vi "host_read_VISA.vi"() -> ()   [LabVIEW 2019]
uses:
  Program Files (x86)/National Instruments/LabVIEW 2019/examples/Instrument IO/Serial/support/Serial - Settings.ctl
  <vilib>/Platform/TimedLoop/XDataNode/timing_clust.ctl
  <vilib>/Platform/TimedLoop/XDataNode/nitl_modes.ctl
  <vilib>/Platform/TimedLoop/XDataNode/wakeup.ctl
  <vilib>/Instr/_visa.llb/VISA Configure Serial Port (Instr).vi
  <vilib>/Utility/file.llb/Write Delimited Spreadsheet (string).vi
  <vilib>/platform/TimedLoop/XDataNode/XDataNode.xnode
  <vilib>/Platform/TimedLoop/XDataNode/XDNodeRunTimeDep.lvlib
panel:
  in  "Data Read Period (ms)":i64=5
  out "data to write":string[](array[string])
  out "Date Formatted with Milliseconds":string
  out "LabVIEW TimeStamp":timestamp
  in  "file path (dialog if empty)":path=path "C:/Users/steve/Dropbox (MIT)/PhD Research/GPASS 2/Electronics/GPASS2-Electronics/Labview/GPASS 2/Data Files/serial/iros_serial.csv"
  in  "Channel Names":string[](array[string])=["Channel 1", "Channel 2", "Channel 3", "Channel 4", "Channel 5"]
  in  "Header Info":string[][](array[string])=[["Test Name", "Operator", "UUT"], ["Voltage", "National Instruments", "AA123"]]
  out "error out":errorcluster
  in  "stop":bool
  in  "End Read on Termination Character?":bool=TRUE
  in  "Serial Settings (read)":T1={"baud rate"=115200, "data bits"=8, "parity"=enum."None", "stop bits"=10, "flow control"=0} {"flow control" items=["None"=0, "XON/XOFF"=1, "RTS/CTS"=2, "DTR/DSR"=4]; "stop bits" items=["1.0"=10, "1.5"=15, "2.0"=20]; "data bits" min=5 max=8 step=1; "baud rate" items=["75"=75, "110"=110, "134"=134, "150"=150, "300"=300, "600"=600, "1200"=1200, "1800"=1800, "2400"=2400, "4800"=4800, "7200"=7200, "9600"=9600, "14400"=14400, "19200"=19200, "28800"=28800, "38400"=38400, "56000"=56000, "57600"=57600, "115200"=115200, "128000"=128000, "230400"=230400]}
  in  "VISA Resource (read)":refnum<visa-resource-name>="COM3"
  out "Read String":string
  out "bytes read":u32
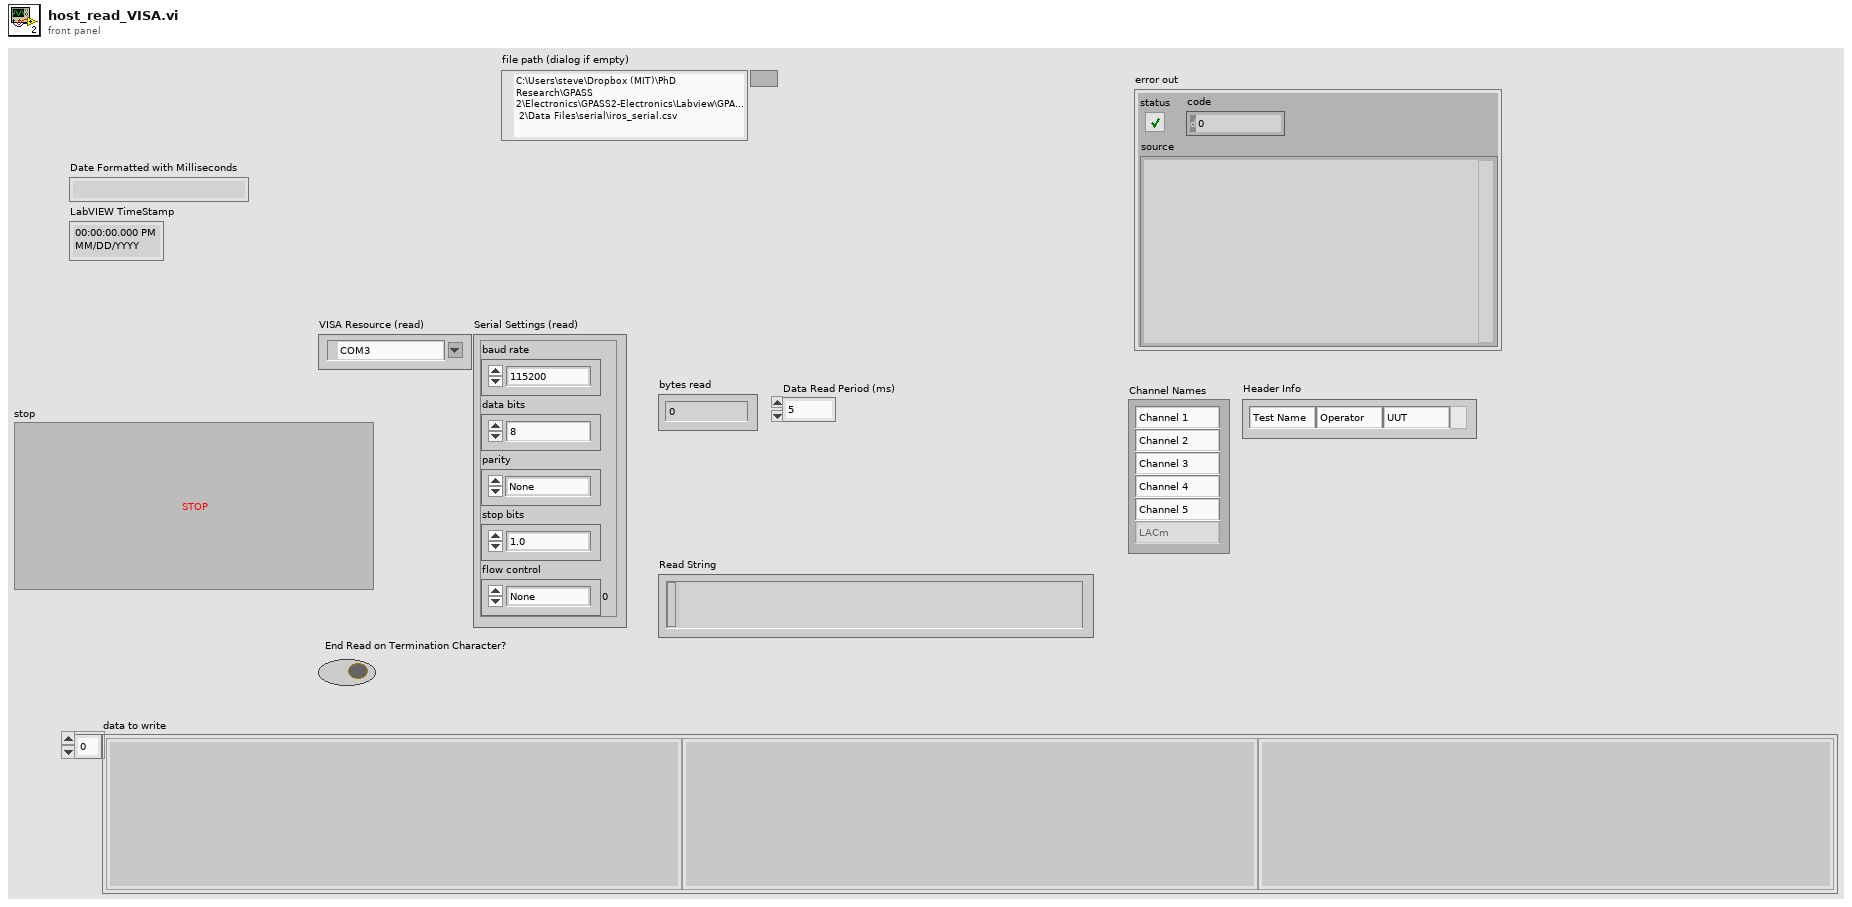
[diagram p1: front panel]
types:
  T1 = typedef "Serial - Settings.ctl" = cluster{"baud rate":u32, "data bits":u16, "parity":enum16{"None", "Odd", "Even", "Mark", "Space"}, "stop bits":u16, "flow control":u16}
  T2 = typedef "XDNodeRunTimeDep.lvlib/timing_clust.ctl" = cluster{"Expected End [f-1]":u64, "Actual End [f-1]":u64, "Finished Late? [f-1]":bool, "Expected End [i-1]":u64, "Actual End [i-1]":u64, "Finished Late? [i-1]":bool, "Expected Start [i]":u64, "Actual Start [i]":u64, "Expected Start [f]":u64, "Actual Start [f]":u64, "Source Name":string, "Structure Name":string, "Period":i64, "Deadline":i64, "Offset":i64, "Start":i64, "Priority":i32, "Timeout":i32, "Mode":T3, "Wakeup Reason":T4, "Error":errorcluster, "Source Type":string, "Secondary Source Type":string, "Global End Time":u64, "Global Start Time":u64, "Frame Duration":u64, "Iteration Duration":u64, "Assigned CPU":i32, "I/O Scan Engine Mode":u32}
  T3 = typedef "XDNodeRunTimeDep.lvlib/nitl_modes.ctl" = enum32{"No Change", "Process missed periods, maintain original phase", "Discard missed periods, maintain original phase", "Process missed periods, ignore original phase", "Discard missed periods, ignore original phase"}
  T4 = typedef "XDNodeRunTimeDep.lvlib/wakeup.ctl" = enum32{"Normal", "Aborted", "Asynchronous wakeup", "Timing source error", "Timed loop error", "Timeout"}
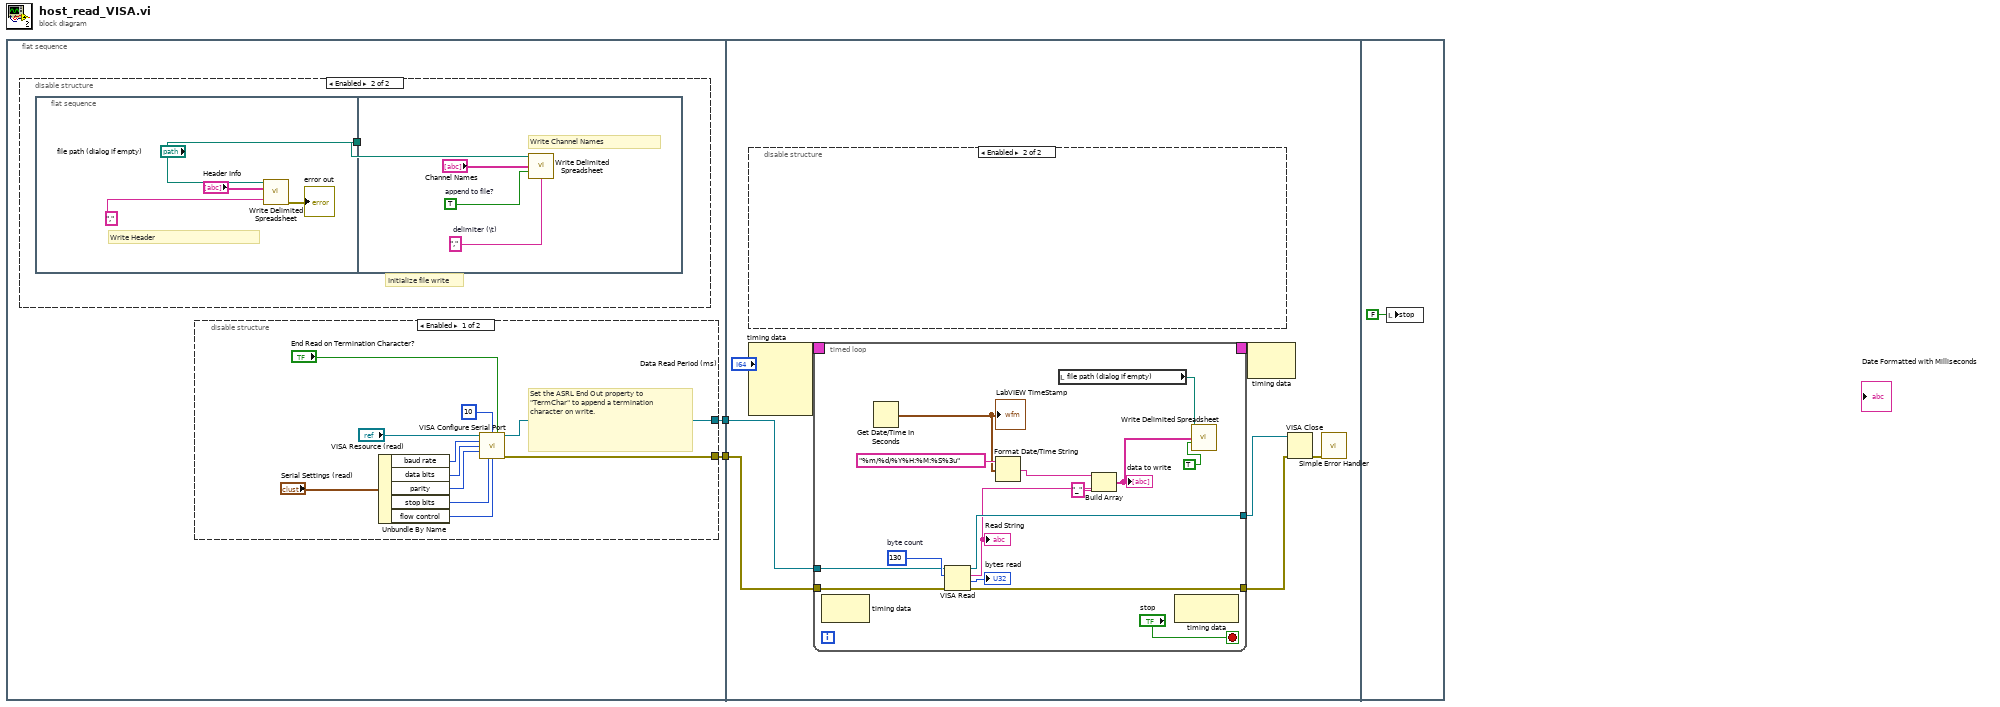
[diagram p0: block diagram]
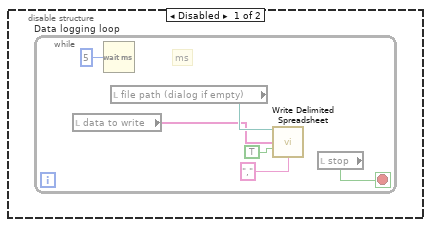
[diagram p4: hidden frame]
diagram:
  n1 = flat-sequence {
    tunnel: [w4] -> w2
    tunnel: [w3] -> w1
    tunnel: w2 -> [w27]
    tunnel: w1 -> [w26]
    frame #0 {
      n2 = disable-structure shown="Enabled" {
        frame Disabled {
        }
        frame Enabled {
          # "Initialize file write"
          n3 = flat-sequence {
            tunnel: ["file path (dialog if empty)"] -> w5
            tunnel: w5 -> [w10]
            frame #0 {
              # "Write Header"
              n4 = call-poly <vilib>:"Write Delimited Spreadsheet.vi"("file path (dialog if empty)"="file path (dialog if empty)", "2D data"="Header Info", "delimiter (\\t)"="," ("delimiter (\\t)")) -> ("error out"=→"error out":errorcluster)  [unwired: 11 in, 1 out]
            }
            frame #1 {
              w12 = TRUE  # append to file?
              w11 = ","  # delimiter (\t)
              # "Write Channel Names"
              n5 = call-poly <vilib>:"Write Delimited Spreadsheet.vi"("file path (dialog if empty)"=w10, "1D data"="Channel Names", "append to file? (new file:F)"=w12, "delimiter (\\t)"=w11) -> ()  [unwired: 10 in, 2 out]
            }
          }
        }
      }
      n6 = disable-structure shown="Enabled" {
        disable-tunnel: [w16 _] -> w4
        disable-tunnel: [w15 _] -> w3
        frame Enabled {
          # "Set the ASRL End Out property to \"TermChar\" to append a termination character on write."
          n7 = Unbundle By Name("Serial Settings (read)") -> ("baud rate"=w22:u32, "data bits"=w21:u16, "parity"=w20:enum16{"None", "Odd", "Even", "Mark", "Space"}, "stop bits"=w19:u16, "flow control"=w18:u16)
          n8 = call-poly "VISA Configure Serial Port"("VISA resource name"="VISA Resource (read)", "termination char\n(0xA = '\\n' = LF)"=u8 10 ("termination char\n(0xA = '\\n' = LF)"), "Enable Termination\nChar (T)"="End Read on Termination Character?", "baud rate (9600)"=w22, "data bits (8)"=w21, "parity (0:none)"=w20, "stop bits (10: 1 bit)"=w19, "flow control (0:none)"=w18) -> ("VISA resource name out"=w16:refnum<visa-resource-name>, "error out"=w15:errorcluster)  [unwired: 2 in, 4 out]
        }
        frame Disabled {
        }
      }
    }
    frame #1 {
      n9 = disable-structure shown="Enabled" {
        frame Disabled {
          n10 = while "Data logging loop" {
            stop <- w37 stop-if-true
            # "ms"
            n11 = local read "data to write"() -> (w33:string[])
            n12 = Wait (ms)(milliseconds to wait=u32 5) -> ()  [unwired: 1 out]
            n13 = local read "file path (dialog if empty)"() -> (w34:path)
            n14 = call-poly <vilib>:"Write Delimited Spreadsheet.vi"("file path (dialog if empty)"=w34, "1D data"=w33, "append to file? (new file:F)"=TRUE, "delimiter (\\t)"="," ("delimiter (\\t)")) -> ()  [unwired: 10 in, 2 out]
            n15 = local read "stop"() -> (w37:bool)
          }
        }
        frame Enabled {
        }
      }
      n16 = node-c288("Data Read Period (ms)") -> (w32:T2)  [unwired: 3 in]
      n17 = timed-loop {
        timing: w32 -> [_]
        timing-out: [_] -> w31
        tunnel: [w51] -> w29
        tunnel: [w50] -> w30
        tunnel: w27 -> [w48]
        tunnel: w26 -> [w47]
        stop <- "stop" stop-if-true
        w53 = u32 130  # byte count
        n18 = node-c288() -> ()  [unwired: 1 in, 1 out]
        n19 = Get Date/Time In Seconds() -> (seconds since 1Jan1904=w45:timestamp)
        "LabVIEW TimeStamp" <- w45
        n20 = VISA Read(VISA resource name=w48, byte count=w53, error in (no error)=w47) -> (VISA resource name out=w51:refnum<visa-resource-name>, read buffer=w43:string, return count=→"bytes read":u32, error out=w50:errorcluster)
        "Read String" <- w43
        n21 = Format Date/Time String(time format string (%c)="%m/%d/%Y%H:%M:%S%3u", seconds (now)=w45) -> (date/time string=w44:string)  [unwired: 1 in]
        n22 = local read "file path (dialog if empty)"() -> (w40:path)
        n23 = Build Array(w44, "_" ("element"), w43) -> (w41:string[])
        "data to write" <- w41
        n24 = node-c288() -> ()  [unwired: 1 in, 1 out]
        n25 = call-poly <vilib>:"Write Delimited Spreadsheet.vi"("file path (dialog if empty)"=w40, "1D data"=w41, "append to file? (new file:F)"=TRUE) -> ()  [unwired: 11 in, 2 out]
      }
      n26 = node-c288(w31) -> ()  [unwired: 1 out]
      n27 = VISA Close(VISA resource name=w29, error in (no error)=w30) -> (error out=w28:errorcluster)
      n28 = call <vilib>:"Simple Error Handler.vi"("error in (no error)"=w28) -> ()  [unwired: 1 in, 8 out]
    }
    frame #2 {
      n29 = local write "stop"(FALSE ("stop")) -> ()
    }
  }
